vi "Exporting VIs - Server.vi"() -> ()   [LabVIEW 2019]
doc: "This is a simple example of a server which exports VIs to be called from another machine. You may run both the client and server on the same machine without modifying the access list. The VIs listed in the Exported VI list are exported by the server."
panel:
  in  "VIs to Export":string[](array[string])
  in  "Stop Server":bool
  # "This is the server VI for the Exporting VIs.vi example. If this VI were running on a remote machine, you could use TCP/IP through VI Server to connect to any Exported VIs that are run by this server. See the block diagram for more information."
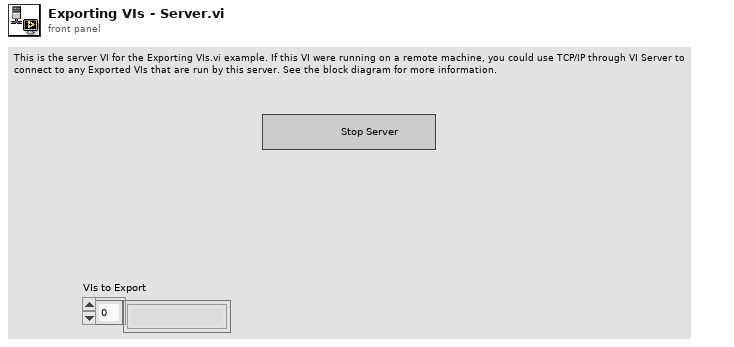
[diagram p1: front panel]
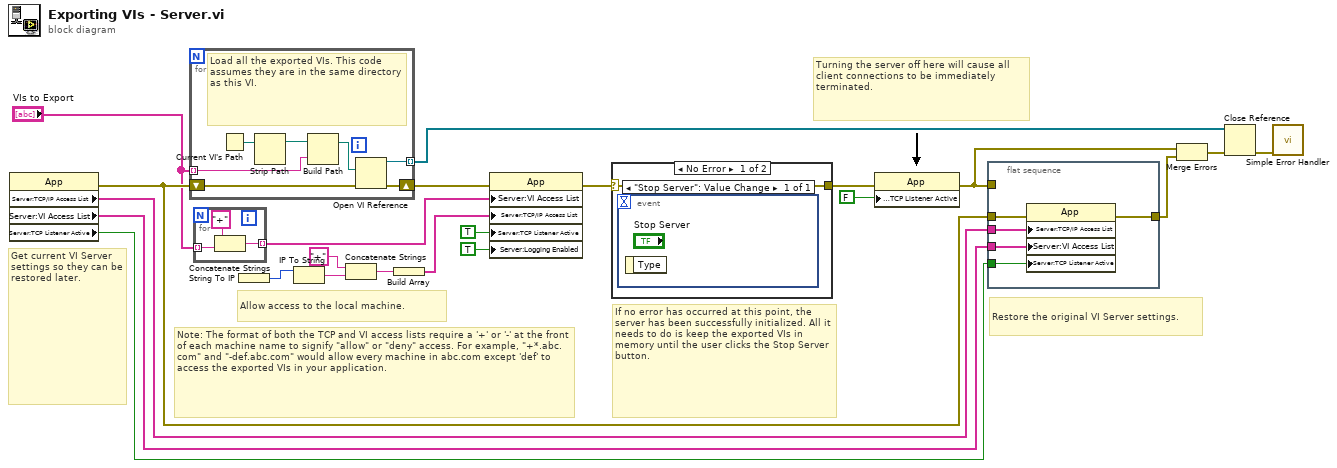
[diagram p0: block diagram]
diagram:
  # "If no error has occurred at this point, the server has been successfully initialized. All it needs to do is keep the exported VIs in memory until the user clicks the Stop Server button."
  # "Restore the original VI Server settings."
  # "Turning the server off here will cause all client connections to be immediately terminated."
  # "Allow access to the local machine."
  # "Note: The format of both the TCP and VI access lists require a '+' or '-' at the front of each machine name to signify \"allow\" or \"deny\" access. For example, \"+*.abc.com\" and \"-def.abc.com\" would allow every machine in abc.com except 'def' to access the exported VIs in your application."
  # "Get current VI Server settings so they can be restored later."
  n1 = property class="App"() -> (error out=w9:errorcluster, "Server:TCP/IP Access List"=w21:string[], "Server:VI Access List"=w22:string[], "Server:TCP Listener Active"=w16:bool)  [unwired: 2 in, 1 out]
  n2 = for {
    tunnel: "VIs to Export" -> [w26] mode=indexing
    tunnel: [w25] -> w3 mode=indexing
    shift-right: [w23] -> w8
    shift-left: w9 -> [w24]
    # "Load all the exported VIs. This code assumes they are in the same directory as this VI."
    n3 = Current VI's Path() -> (path=w29:path)
    n4 = Strip Path(path=w29) -> (stripped path=w27:path)  [unwired: 1 out]
    n5 = Build Path(base path=w27, name or relative path=w26) -> (appended path=w28:path)
    n6 = Open VI Reference(vi path=w28, error in (no error)=w24) -> (vi reference=w25:refnum<vi>, error out=w23:errorcluster)  [unwired: 4 in]
  }
  n7 = for {
    tunnel: "VIs to Export" -> [w32] mode=indexing
    tunnel: [w30] -> w6 mode=indexing
    n8 = Concatenate Strings("+", w32) -> (w30:string)
  }
  n9 = String To IP() -> (0:w20:u32)  [unwired: 1 in]
  n10 = IP To String(2:w20) -> (0:w12:string)  [unwired: 1 in]
  n11 = Concatenate Strings("+", w12) -> (w7:string)
  n12 = Build Array(w7) -> (w10:string[])
  n13 = property class="App"(error in=w8, "Server:VI Access List"=w6, "Server:TCP/IP Access List"=w10, "Server:TCP Listener Active"=TRUE, "Server:Logging Enabled"=TRUE) -> (error out=w2:errorcluster)  [unwired: 1 in, 1 out]
  n14 = case shown="No Error" w2 {
    selector: w2 -> [w33 w34]
    tunnel: [w33 w34] -> w1
    frame No Error {
      n15 = event shown="[0] \"Stop Server\": Value Change" {
        selector: _ -> [_]
        dyn-events: _ -> [_]
        timeout: _ -> [_]
        event "Stop Server": Value Change {
          n16 = event-data() -> ()  [unwired: 1 in, 1 out]
        }
      }
    }
    frame Error {
      # "An error occurred. Do not wait for the user to click the Stop Server button."
    }
  }
  n17 = property class="App"(error in=w1, "Server:TCP Listener Active"=FALSE) -> (error out=w14:errorcluster)  [unwired: 1 in, 1 out]
  n18 = flat-sequence {
    tunnel: w22 -> [w39]
    tunnel: w21 -> [w38]
    tunnel: w16 -> [w37]
    tunnel: w14 -> [_]
    tunnel: [w36] -> w13
    tunnel: w9 -> [w35]
    frame #0 {
      n19 = property class="App"(error in=w35, "Server:TCP/IP Access List"=w38, "Server:VI Access List"=w39, "Server:TCP Listener Active"=w37) -> (error out=w36:errorcluster)  [unwired: 1 in, 1 out]
    }
  }
  n20 = Merge Errors(w14, w13) -> (w15:errorcluster)
  n21 = Close Reference(reference=w3, error in (no error)=w15) -> (error out=w4:errorcluster)
  n22 = call <vilib>:"Simple Error Handler.vi"("error in (no error)"=w4) -> ()  [unwired: 4 in, 5 out]
